vi "DIO.vi"() -> ()   [LabVIEW 2019]
panel:
  in  "Write DO":bool
  out "return":i16
  in  "BaudRate":u32=115200
  out "DO_Readback":u32
  in  "DI_TotalCh":i16=4
  in  "DOTotalCh":i16=4
  in  "DO_Value":u32
  out "DI_Value":u32
  in  "DIO_Module":T1={"ComPort"=1, "Address"=1, "Slot"=1, "CheckSum"=0, "TimeOut"=1000}
  in  "stop":bool
  # "Module setting"
  # "Write DO"
  # "Read status"
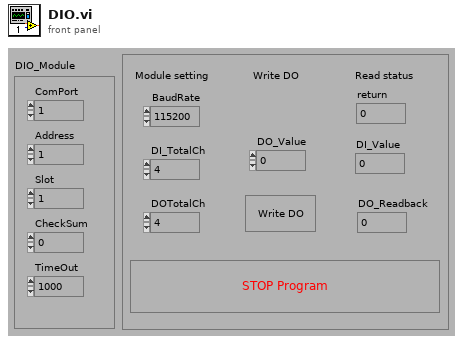
[diagram p1: front panel]
types:
  T1 = cluster{"ComPort":u8, "Address":i16, "Slot":i16, "CheckSum":i16, "TimeOut":i16}
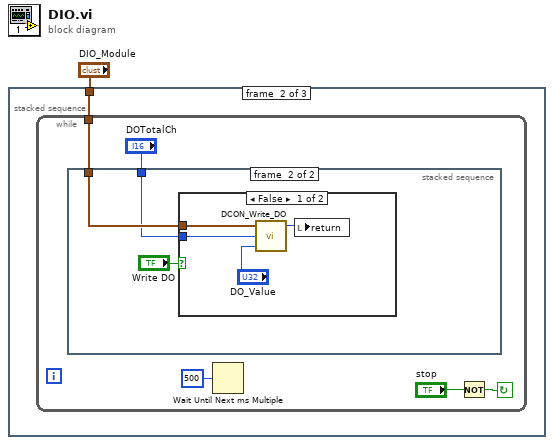
[diagram p0: block diagram]
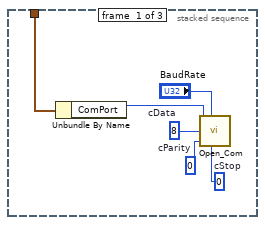
[diagram p2: hidden frame]
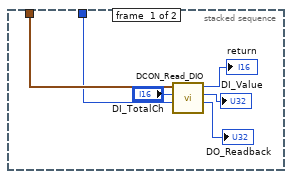
[diagram p3: hidden frame]
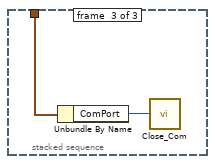
[diagram p5: hidden frame]
diagram:
  n1 = stacked-sequence {
    tunnel: "DIO_Module" -> [w4 w8 w28]
    frame #0 {
      w5 = u8 0  # cStop
      w6 = u8 0  # cParity
      w7 = u8 8  # cData
      n2 = Unbundle By Name(w4) -> ("ComPort"=w3:u8)
      n3 = call "Open_Com.VI"("port number"=w3, "baudrate (115200)"="BaudRate", "data bit (8)"=w7, "parity (0: none)"=w6, "stop bit (0: 1 stop bit)"=w5) -> ()  [unwired: 1 out]
    }
    frame #1 {
      n4 = while {
        tunnel: w8 -> [w10]
        stop <- w13 continue-if-true
        n5 = stacked-sequence {
          tunnel: w10 -> [w18 w22]
          tunnel: "DOTotalCh" -> [w16 w21]
          frame #0 {
            n6 = call "DCON_Read_DIO.vi"("DO_TotalCh"=w16, "DI_TotalCh"="DI_TotalCh", "DCON_Module"=w18) -> ("DO_Value"=→"DO_Readback":u32, "DI_Value"=→"DI_Value":u32, "return"=→"return":i16)  [unwired: 2 out]
          }
          frame #1 {
            n7 = case shown="False" "Write DO" {
              tunnel: w22 -> [w25 _]
              tunnel: w21 -> [w24 _]
              frame False {
                n8 = call "DCON_Write_DO.vi"("DO_Value"="DO_Value", "DOTotalCh"=w24, "DCON_Module"=w25) -> ("return"=w23:i16)  [unwired: 2 in]
                n9 = local write "return"(w23) -> ()
              }
              frame True {
              }
            }
          }
        }
        n10 = Wait Until Next ms Multiple(millisecond multiple=u32 500) -> ()  [unwired: 1 out]
        n11 = Not(x="stop") -> (.not. x?=w13:bool)
      }
    }
    frame #2 {
      n12 = Unbundle By Name(w28) -> ("ComPort"=w27:u8)
      n13 = call "Close_Com.vi"("port number"=w27) -> ()  [unwired: 1 out]
    }
  }
